vi "Copy Package.vi"(8 "error in (no error)":errorcluster, 9 "Product Name":string, 10 "Output Package File Path":path, 11 "Package Source Folder":path) -> (0 "error out":errorcluster)   [LabVIEW 2016]
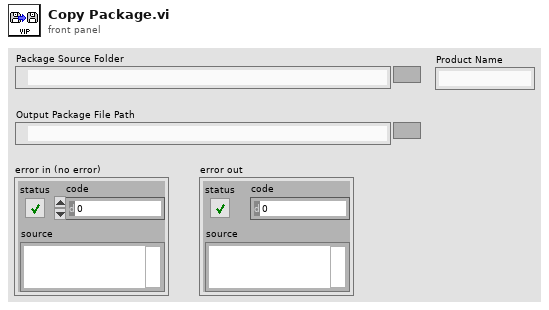
[diagram p1: front panel]
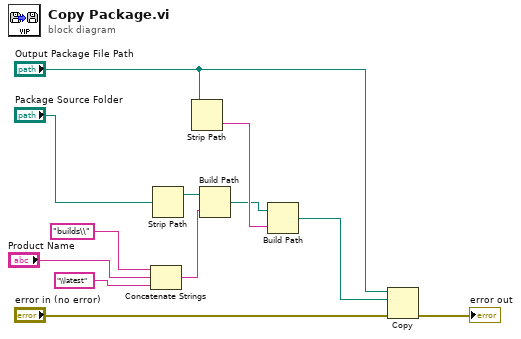
[diagram p0: block diagram]
diagram:
  n1 = Concatenate Strings("builds\\" ("name or relative path"), "Product Name", "\\latest" ("name or relative path")) -> (w1:string)
  n2 = Strip Path(path="Package Source Folder") -> (stripped path=w10:path)  [unwired: 1 out]
  n3 = Strip Path(path="Output Package File Path") -> (name=w8:string)  [unwired: 1 out]
  n4 = Build Path(base path=w10, name or relative path=w1) -> (appended path=w5:path)
  n5 = Build Path(base path=w5, name or relative path=w8) -> (appended path=w7:path)
  n6 = Copy(8:"error in (no error)", 10:w7, 11:"Output Package File Path") -> (0:→"error out":errorcluster)  [unwired: 2 in, 2 out]
